vi "Decode.vi"(11 "Encoded  File":path) -> (2 "array":string[][](array[string]), 3 "Decoded File":path)   [LabVIEW 2022 SP3]
uses:
  <vilib>/Utility/file.llb/Read Delimited Spreadsheet (string).vi
  <vilib>/Utility/file.llb/Write Delimited Spreadsheet (string).vi
panel:
  out "Decoded Value":string
  in  "error IO":errorcluster
  out "Encoded Value":string
  # "DECODE"
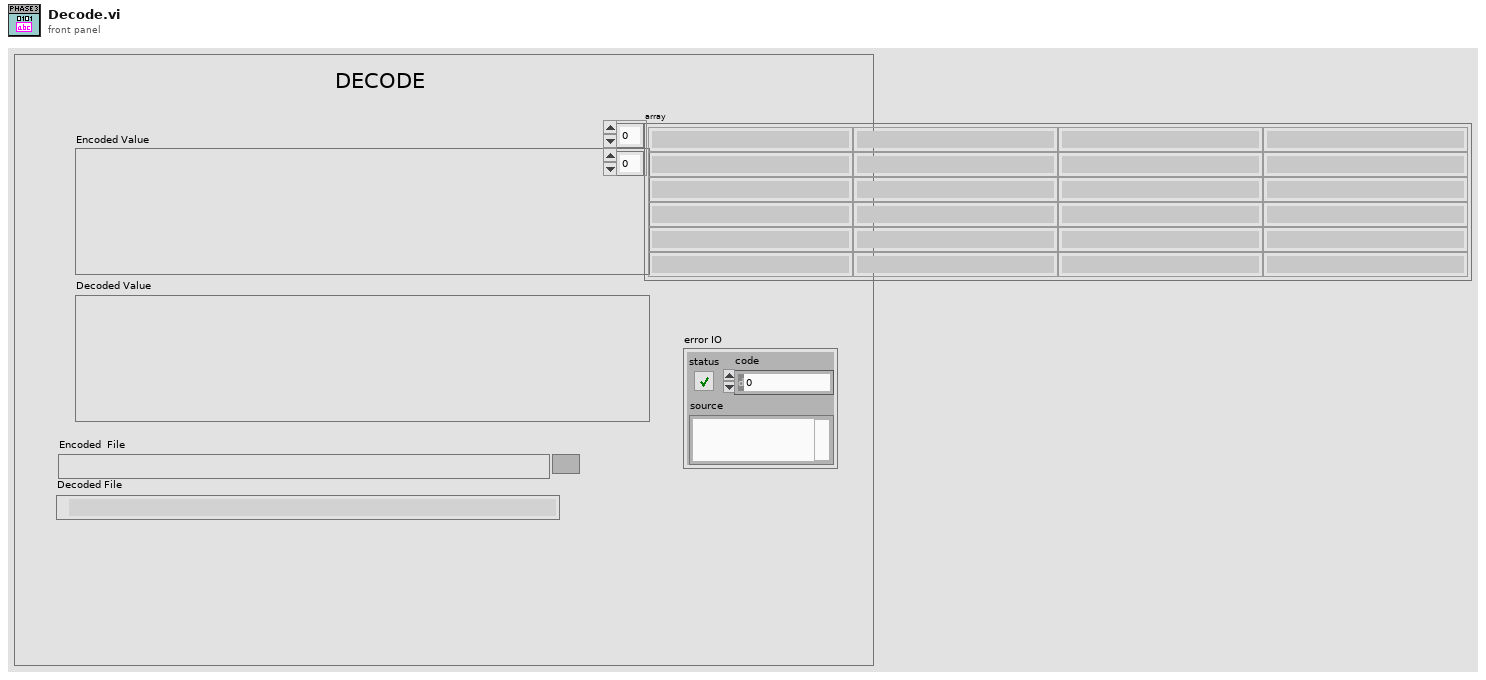
[diagram p1: front panel]
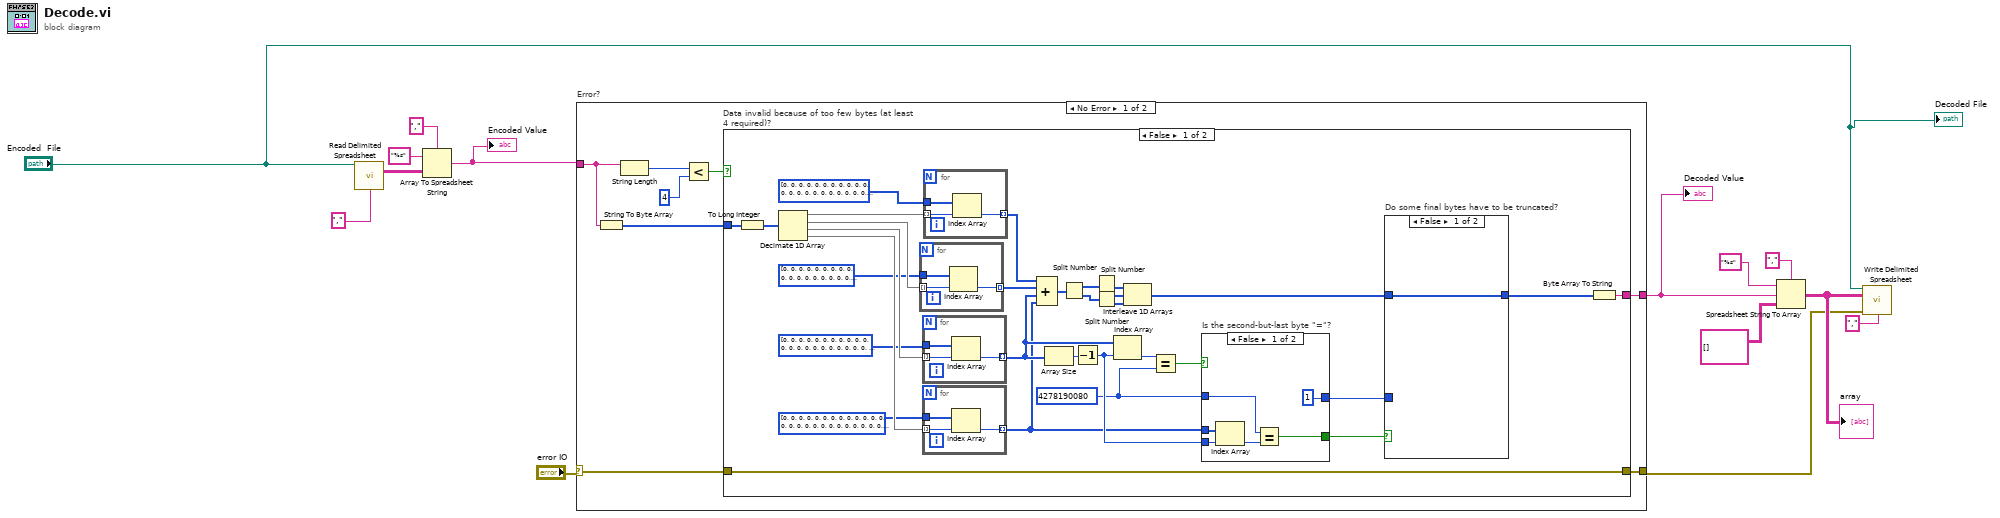
[diagram p0: block diagram]
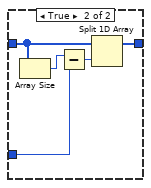
[diagram p2: hidden frame]
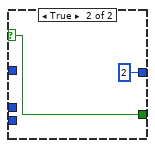
[diagram p3: hidden frame]
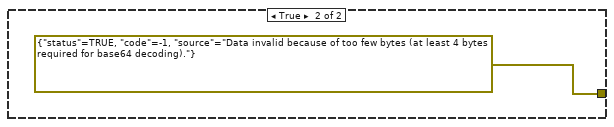
[diagram p4: hidden frame]
diagram:
  n1 = call-poly <vilib>:"Read Delimited Spreadsheet.vi"("file path (dialog if empty)"="Encoded  File", "delimiter (\\t)"="," ("delimiter (\\t)")) -> ("all rows"=w9:string[][])  [unwired: 8 in, 5 out]
  n2 = Array To Spreadsheet String(delimiter (Tab)=",", array=w9, 3:"%s" ("format string")) -> (spreadsheet string=w5:string)
  "Encoded Value" <- w5
  n3 = case "Error?" shown="No Error" "error IO" {
    selector: "error IO" -> [w17 w81]
    tunnel: w5 -> [w21 _]
    tunnel: [w16 w81] -> w4
    tunnel: [w15 _] -> w2
    frame No Error {
      n4 = String To Byte Array(string=w21) -> (unsigned byte array=w20:u8[])
      n5 = String Length(string=w21) -> (length=w18:i32)
      n6 = Less?(x=w18, y=4) -> (x < y?=w19:bool)
      n7 = case "Data invalid because of too few bytes (at least 4 required)?" shown="False" w19 {
        tunnel: w20 -> [w35 _]
        tunnel: [w53 _] -> w15
        tunnel: [w23 errorcluster {"status"=TRUE, "code"=-1, "source"="Data invalid because of too few bytes (at least 4 bytes required for base64 decoding)."} ("error IO")] -> w16
        tunnel: w17 -> [w23 _]
        frame False {
          w28 = u32 4278190080 ("y")
          n8 = To Long Integer(number=w35) -> (32bit integer=w52:i32[])
          n9 = Decimate 1D Array(w52) -> (w41:i32[], w51:i32[], w42:i32[], w40:i32[])
          n10 = for {
            tunnel: w51 -> [w75] mode=indexing
            tunnel: u32[] [0, 0, 0, 0, 0, 0, 0, 0, 0, 0, 0, 0, 0, 0, 0, 0, 0, 0, 0, 0, 0, 0, 0, 0, 0, 0, 0, 0, 0, 0, 0, 0, 0, 0, 0, 0, 0, 0, 0, 0, 0, 0, 0, 253952, 0, 0, 0, 258048, 212992, 217088, 221184, 225280, 229376, 233472, 237568, 241664, 245760, 249856, 0, 0, 0, 0, 0, 0, 0, 0, 4096, 8192, 12288, 16384, 20480, 24576, 28672, 32768, 36864, 40960, 45056, 49152, 53248, 57344, 61440, 65536, 69632, 73728, 77824, 81920, 86016, 90112, 94208, 98304, 102400, 0, 0, 0, 0, 0, 0, 106496, 110592, 114688, 118784, 122880, 126976, 131072, 135168, 139264, 143360, 147456, 151552, 155648, 159744, 163840, 167936, 172032, 176128, 180224, 184320, 188416, 192512, 196608, 200704, 204800, 208896, 0, 0, 0, 0, 0, 0, 0, 0, 0, 0, 0, 0, 0, 0, 0, 0, 0, 0, 0, 0, 0, 0, 0, 0, 0, 0, 0, 0, 0, 0, 0, 0, 0, 0, 0, 0, 0, 0, 0, 0, 0, 0, 0, 0, 0, 0, 0, 0, 0, 0, 0, 0, 0, 0, 0, 0, 0, 0, 0, 0, 0, 0, 0, 0, 0, 0, 0, 0, 0, 0, 0, 0, 0, 0, 0, 0, 0, 0, 0, 0, 0, 0, 0, 0, 0, 0, 0, 0, 0, 0, 0, 0, 0, 0, 0, 0, 0, 0, 0, 0, 0, 0, 0, 0, 0, 0, 0, 0, 0, 0, 0, 0, 0, 0, 0, 0, 0, 0, 0, 0, 0, 0, 0, 0, 0, 0, 0, 0, 0, 0, 0, 0, 0] ("array 3") -> [w76]
            tunnel: [w74] -> w49 mode=indexing
            n11 = Index Array(array=w76, index=w75) -> (element=w74:u32)
          }
          n12 = for {
            tunnel: u32[] [0, 0, 0, 0, 0, 0, 0, 0, 0, 0, 0, 0, 0, 0, 0, 0, 0, 0, 0, 0, 0, 0, 0, 0, 0, 0, 0, 0, 0, 0, 0, 0, 0, 0, 0, 0, 0, 0, 0, 0, 0, 0, 0, 3968, 0, 0, 0, 4032, 3328, 3392, 3456, 3520, 3584, 3648, 3712, 3776, 3840, 3904, 0, 0, 0, 4278190080, 0, 0, 0, 0, 64, 128, 192, 256, 320, 384, 448, 512, 576, 640, 704, 768, 832, 896, 960, 1024, 1088, 1152, 1216, 1280, 1344, 1408, 1472, 1536, 1600, 0, 0, 0, 0, 0, 0, 1664, 1728, 1792, 1856, 1920, 1984, 2048, 2112, 2176, 2240, 2304, 2368, 2432, 2496, 2560, 2624, 2688, 2752, 2816, 2880, 2944, 3008, 3072, 3136, 3200, 3264, 0, 0, 0, 0, 0, 0, 0, 0, 0, 0, 0, 0, 0, 0, 0, 0, 0, 0, 0, 0, 0, 0, 0, 0, 0, 0, 0, 0, 0, 0, 0, 0, 0, 0, 0, 0, 0, 0, 0, 0, 0, 0, 0, 0, 0, 0, 0, 0, 0, 0, 0, 0, 0, 0, 0, 0, 0, 0, 0, 0, 0, 0, 0, 0, 0, 0, 0, 0, 0, 0, 0, 0, 0, 0, 0, 0, 0, 0, 0, 0, 0, 0, 0, 0, 0, 0, 0, 0, 0, 0, 0, 0, 0, 0, 0, 0, 0, 0, 0, 0, 0, 0, 0, 0, 0, 0, 0, 0, 0, 0, 0, 0, 0, 0, 0, 0, 0, 0, 0, 0, 0, 0, 0, 0, 0, 0, 0, 0, 0, 0, 0, 0, 0] ("array 2") -> [w73]
            tunnel: [w72] -> w33 mode=indexing
            tunnel: w42 -> [w71] mode=indexing
            n13 = Index Array(array=w73, index=w71) -> (element=w72:u32)
          }
          n14 = for {
            tunnel: u32[] [0, 0, 0, 0, 0, 0, 0, 0, 0, 0, 0, 0, 0, 0, 0, 0, 0, 0, 0, 0, 0, 0, 0, 0, 0, 0, 0, 0, 0, 0, 0, 0, 0, 0, 0, 0, 0, 0, 0, 0, 0, 0, 0, 62, 0, 0, 0, 63, 52, 53, 54, 55, 56, 57, 58, 59, 60, 61, 0, 0, 0, 4278190080, 0, 0, 0, 0, 1, 2, 3, 4, 5, 6, 7, 8, 9, 10, 11, 12, 13, 14, 15, 16, 17, 18, 19, 20, 21, 22, 23, 24, 25, 0, 0, 0, 0, 0, 0, 26, 27, 28, 29, 30, 31, 32, 33, 34, 35, 36, 37, 38, 39, 40, 41, 42, 43, 44, 45, 46, 47, 48, 49, 50, 51, 0, 0, 0, 0, 0, 0, 0, 0, 0, 0, 0, 0, 0, 0, 0, 0, 0, 0, 0, 0, 0, 0, 0, 0, 0, 0, 0, 0, 0, 0, 0, 0, 0, 0, 0, 0, 0, 0, 0, 0, 0, 0, 0, 0, 0, 0, 0, 0, 0, 0, 0, 0, 0, 0, 0, 0, 0, 0, 0, 0, 0, 0, 0, 0, 0, 0, 0, 0, 0, 0, 0, 0, 0, 0, 0, 0, 0, 0, 0, 0, 0, 0, 0, 0, 0, 0, 0, 0, 0, 0, 0, 0, 0, 0, 0, 0, 0, 0, 0, 0, 0, 0, 0, 0, 0, 0, 0, 0, 0, 0, 0, 0, 0, 0, 0, 0, 0, 0, 0, 0, 0, 0, 0, 0, 0, 0, 0, 0, 0, 0, 0, 0, 0] ("Array") -> [w70]
            tunnel: [w69] -> w31 mode=indexing
            tunnel: w40 -> [w68] mode=indexing
            n15 = Index Array(array=w70, index=w68) -> (element=w69:u32)
          }
          n16 = for {
            tunnel: w41 -> [w78] mode=indexing
            tunnel: u32[] [0, 0, 0, 0, 0, 0, 0, 0, 0, 0, 0, 0, 0, 0, 0, 0, 0, 0, 0, 0, 0, 0, 0, 0, 0, 0, 0, 0, 0, 0, 0, 0, 0, 0, 0, 0, 0, 0, 0, 0, 0, 0, 0, 16252928, 0, 0, 0, 16515072, 13631488, 13893632, 14155776, 14417920, 14680064, 14942208, 15204352, 15466496, 15728640, 15990784, 0, 0, 0, 0, 0, 0, 0, 0, 262144, 524288, 786432, 1048576, 1310720, 1572864, 1835008, 2097152, 2359296, 2621440, 2883584, 3145728, 3407872, 3670016, 3932160, 4194304, 4456448, 4718592, 4980736, 5242880, 5505024, 5767168, 6029312, 6291456, 6553600, 0, 0, 0, 0, 0, 0, 6815744, 7077888, 7340032, 7602176, 7864320, 8126464, 8388608, 8650752, 8912896, 9175040, 9437184, 9699328, 9961472, 10223616, 10485760, 10747904, 11010048, 11272192, 11534336, 11796480, 12058624, 12320768, 12582912, 12845056, 13107200, 13369344, 0, 0, 0, 0, 0, 0, 0, 0, 0, 0, 0, 0, 0, 0, 0, 0, 0, 0, 0, 0, 0, 0, 0, 0, 0, 0, 0, 0, 0, 0, 0, 0, 0, 0, 0, 0, 0, 0, 0, 0, 0, 0, 0, 0, 0, 0, 0, 0, 0, 0, 0, 0, 0, 0, 0, 0, 0, 0, 0, 0, 0, 0, 0, 0, 0, 0, 0, 0, 0, 0, 0, 0, 0, 0, 0, 0, 0, 0, 0, 0, 0, 0, 0, 0, 0, 0, 0, 0, 0, 0, 0, 0, 0, 0, 0, 0, 0, 0, 0, 0, 0, 0, 0, 0, 0, 0, 0, 0, 0, 0, 0, 0, 0, 0, 0, 0, 0, 0, 0, 0, 0, 0, 0, 0, 0, 0, 0, 0, 0, 0, 0, 0, 0] ("array 4") -> [w79]
            tunnel: [w77] -> w50 mode=indexing
            n17 = Index Array(array=w79, index=w78) -> (element=w77:u32)
          }
          n18 = Compound Arithmetic op=ADD(w50, w49, w33, w31) -> (w47:u32[])
          n19 = Array Size(array=w33) -> (size(s)=w34:i32)
          n20 = Split Number(x=w47) -> (hi(x)=w48:u16[], lo(x)=w46:u16[])
          n21 = Decrement(x=w34) -> (x-1=w32:i32)
          n22 = Split Number(x=w48) -> (lo(x)=w43:u8[])  [unwired: 1 out]
          n23 = Split Number(x=w46) -> (hi(x)=w44:u8[], lo(x)=w45:u8[])
          n24 = Index Array(array=w33, index=w32) -> (element=w30:u32)
          n25 = Interleave 1D Arrays(w43, w44, w45) -> (w25:u8[])
          n26 = Equal?(x=w30, y=w28) -> (x = y?=w29:bool)
          n27 = case "Is the second-but-last byte \"=\"?" shown="False" w29 {
            selector: w29 -> [_ w66]
            tunnel: w32 -> [w65 _]
            tunnel: w31 -> [w64 _]
            tunnel: w28 -> [w62 _]
            tunnel: [w61 w66] -> w27
            tunnel: [1 2] -> w26
            frame False {
              n28 = Index Array(array=w64, index=w65) -> (element=w63:u32)
              n29 = Equal?(x=w62, y=w63) -> (x = y?=w61:bool)
            }
            frame True {
            }
          }
          n30 = case "Do some final bytes have to be truncated?" shown="False" w27 {
            tunnel: w26 -> [_ w59]
            tunnel: w25 -> [w54 w55]
            tunnel: [w54 w57] -> w24
            frame False {
            }
            frame True {
              n31 = Array Size(array=w55) -> (size(s)=w56:i32)
              n32 = Subtract(x=w56, y=w59) -> (x-y=w58:i32)
              n33 = Split 1D Array(array=w55, index=w58) -> (first subarray=w57:u8[])  [unwired: 1 out]
            }
          }
          n34 = Byte Array To String(unsigned byte array=w24) -> (string=w53:string)
        }
        frame True {
        }
      }
    }
    frame Error {
    }
  }
  "Decoded Value" <- w2
  n35 = Spreadsheet String To Array(delimiter (Tab)=",", format string="%s", spreadsheet string=w2, array type (2D Dbl)=string[][] [] ("all rows")) -> (array=w12:string[][])
  "array" <- w12
  n36 = call-poly <vilib>:"Write Delimited Spreadsheet.vi"("file path (dialog if empty)"="Encoded  File", "2D data"=w12, "error in (no error)"=w4, "delimiter (\\t)"="," ("delimiter (\\t)")) -> ()  [unwired: 10 in, 2 out]
  "Decoded File" <- "Encoded  File"
